vi "XYZ Stage-Cleanup (ver 2).vi"(8 "error in (no error)":errorcluster, 11 "XYZ Stage Control in":refnum<class "XYZ Stage Control.lvclass">) -> (0 "error out":errorcluster, 3 "XYZ Stage Control out":refnum<class "XYZ Stage Control.lvclass">)   [LabVIEW 2020]
uses:
  XYZ Stage Control/XYZ Stage Control.lvclass
  <vilib>/Utility/error.llb/DialogType.ctl
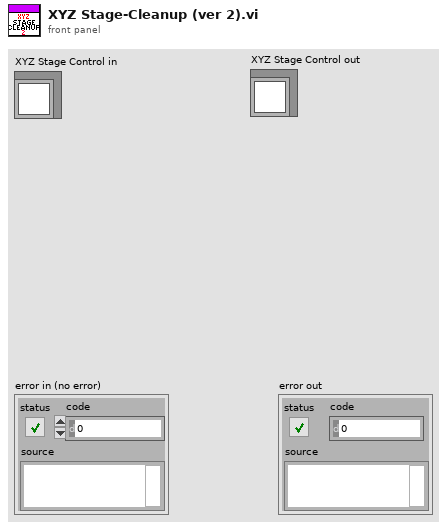
[diagram p1: front panel]
types:
  T1 = typedef "DialogType.ctl" = u16
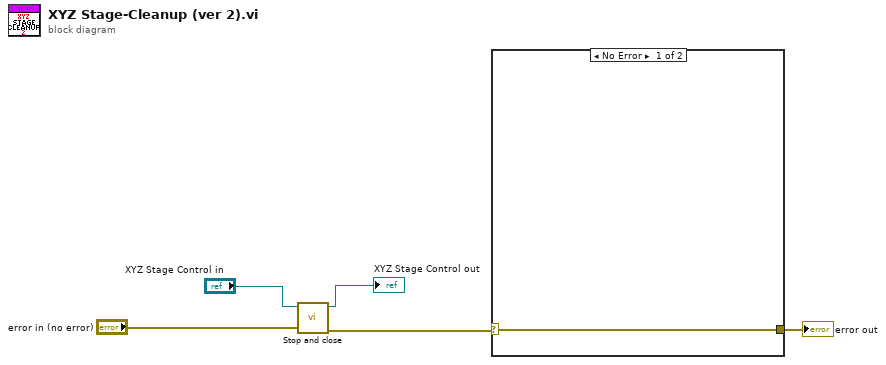
[diagram p0: block diagram]
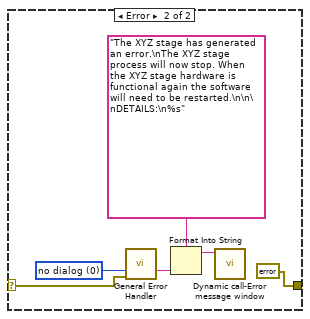
[diagram p2: hidden frame]
diagram:
  n1 = call-dynamic "Stop and close.vi"("error in (no error)"="error in (no error)", "XYZ Stage Control in"="XYZ Stage Control in") -> ("error out"=w3:errorcluster, "XYZ Stage Control out"=→"XYZ Stage Control out":refnum<class "XYZ Stage Control.lvclass">)  [unwired: 8 in]
  n2 = case shown="No Error" w3 {
    selector: w3 -> [w6 w8]
    tunnel: [w6 errorcluster {"status"=FALSE, "code"=0, "source"=""} ("error out")] -> w5
    frame No Error {
    }
    frame Error {
      w10 = T1 0 items=["no dialog", "OK message", "continue or stop message", "OK message + warnings", "continue/stop + warnings"] ("type of dialog (OK msg:1)")
      n3 = call <vilib>:"General Error Handler.vi"("type of dialog (OK msg:1)"=w10, "error in (no error)"=w8) -> ("message"=w9:string)  [unwired: 9 in, 4 out]
      n4 = Format Into String(format string="The XYZ stage has generated an error.\nThe XYZ stage process will now stop. When the XYZ stage hardware is functional again the software will need to be restarted.\n\n\nDETAILS:\n%s" ("Error Source"), w9) -> (resulting string=w7:string)  [unwired: 2 in, 1 out]
      n5 = call "Dynamic call-Error message window.vi"("Error Message"=w7) -> ()  [unwired: 10 in, 1 out]
    }
  }
  "error out" <- w5
